vi "generic api send msg GENERIC MESSAGE.vi"(8 "data":variant, 10 "target (thermometer controller)":string="thermometer controller", 11 "sender":string) -> ()   [LabVIEW 2019]
uses:
  common/common data types/common_event_data.ctl
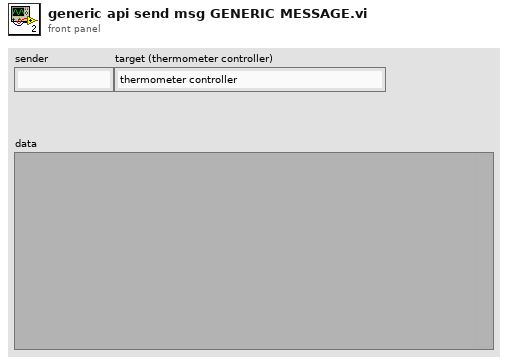
[diagram p1: front panel]
types:
  T1 = typedef "common_event_data.ctl" = cluster{"sender":string, "target":string, "msg":string, "data":variant}
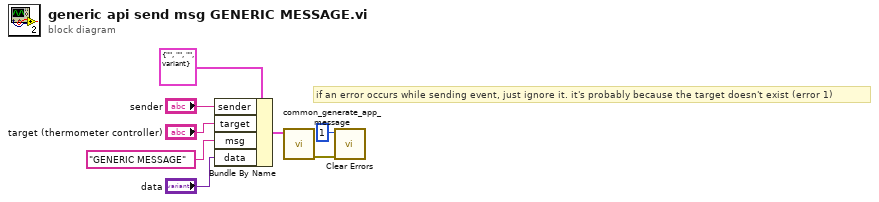
[diagram p0: block diagram]
diagram:
  # "if an error occurs while sending event, just ignore it. it's probably because the target doesn't exist (error 1)"
  n1 = Bundle By Name(cluster=T1 {"sender"="", "target"="", "msg"="", "data"=variant} ("event data"), "sender"="sender", "target"="target (thermometer controller)", "msg"="GENERIC MESSAGE", "data"="data") -> (w8:T1)
  n2 = call "common_generate_app_message.vi"("event data"=w8) -> ("error out"=w2:errorcluster)  [unwired: 10 in]
  n3 = call <vilib>:"Clear Errors.vi"("error in (no error)"=w2, "specific error code to clear (0: all)"=1) -> ()  [unwired: 4 in, 2 out]
